vi "calcDemandedPressureOutputPRamp.vi"(8 "error in (no error)":errorcluster, 9 "loopPeriod":dbl[unit]=5000.0 min=10.0 max=5000.0, 10 "Pressure Valve Opening (%)":dbl=2.0 min=1.0 max=4.0, 11 "SystemController in":refnum<class "SystemController.lvclass">) -> (0 "error out":errorcluster, 2 "rampOutput (%)":dbl=5000.0 min=10.0 max=5000.0, 3 "SystemController out":refnum<class "SystemController.lvclass">)   [LabVIEW 2015, in "SystemController.lvclass"]
uses:
  SystemController.lvclass
  SystemController.lvclass/SystemController.ctl
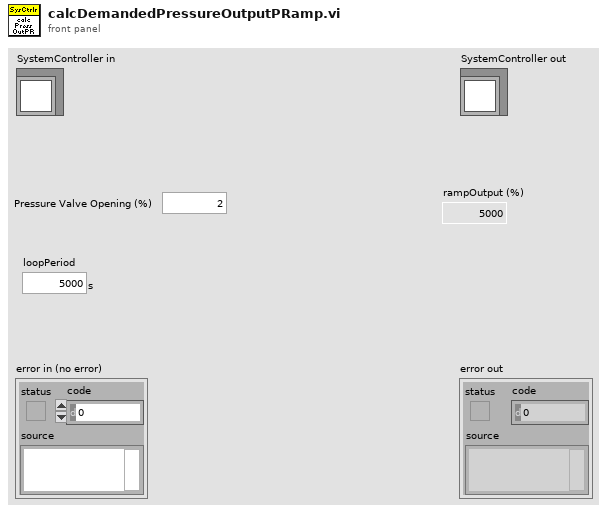
[diagram p1: front panel]
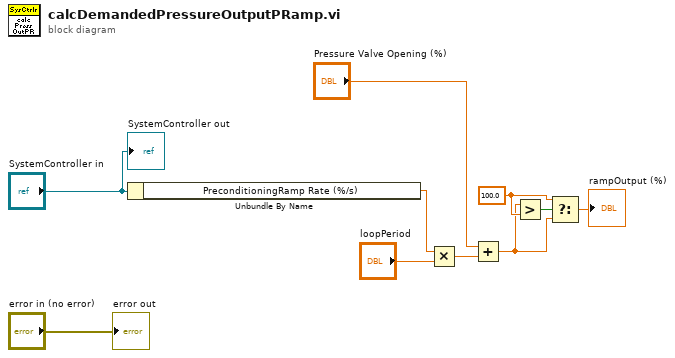
[diagram p0: block diagram]
diagram:
  w3 = 100.0 ("y")
  n1 = Unbundle By Name("SystemController in") -> ("PreconditioningRamp Rate (%/s)"=w8:dbl[unit])
  n2 = Multiply(x=w8, y="loopPeriod") -> (x*y=w6:dbl)
  n3 = Add(x="Pressure Valve Opening (%)", y=w6) -> (x+y=w1:dbl)
  n4 = Greater?(x=w1, y=w3) -> (0:w4:bool)
  n5 = Select(t=w3, s=w4, f=w1) -> (s? t:f=→"rampOutput (%)":dbl)
  "error out" <- "error in (no error)"
  "SystemController out" <- "SystemController in"
